vi "Reverse Camera Orientation.vi"(0 "P1X":dbl[](array[numeric]), 1 "P1Y":dbl[](array[numeric]), 2 "P2X":dbl[](array[numeric]), 3 "P2Y":dbl[](array[numeric]), 4 "P3X":dbl[](array[numeric]), 5 "P3Y":dbl[](array[numeric]), 6 "Apply Transform?":bool, 7 "Calibration Data":T1 {"y" format="%.2f"; "z" format="%.2f"; "theta" format="%.2f"; "phi" format="%.2f"; "d" format="%.2f"}, 8 "Stored Camera Orientation":enum16{"Horizontal", "Vertical"}(ring), 10 "Eye":enum16{"Right", "Left"}(ring)=enum."Left") -> (13 "Calibration Data out":T1 {"y" format="%.2f"; "z" format="%.2f"; "theta" format="%.2f"; "phi" format="%.2f"; "d" format="%.2f"}, 14 "P1X out":dbl[](array[numeric]), 15 "P1Y out":dbl[](array[numeric]), 16 "P2X out":dbl[](array[numeric]), 17 "P2Y out":dbl[](array[numeric]), 18 "P3X out":dbl[](array[numeric]), 19 "P3Y out":dbl[](array[numeric]))   [LabVIEW 2016]
doc: "Author: William Figtree\nDate: 7/02/2016\nDescription:\nVI reverse the camera orientation selected during aquisition by transforming the X and Y pixel coordinates.s"
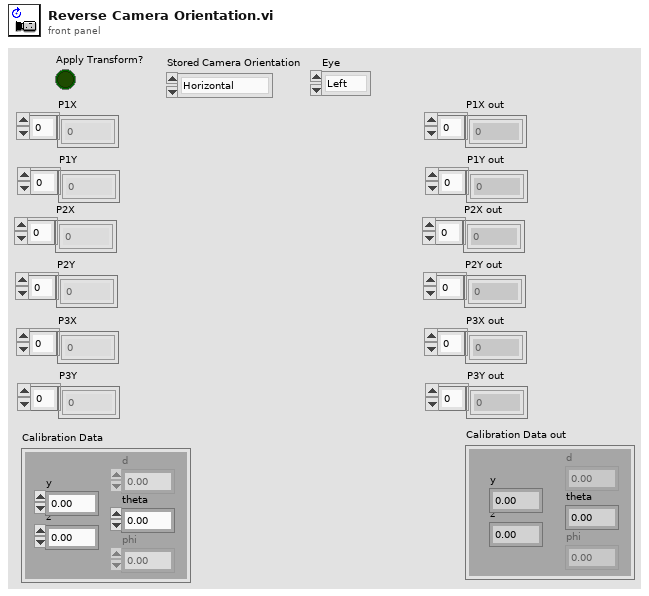
[diagram p1: front panel]
types:
  T1 = cluster{"d":dbl, "phi":dbl, "theta":dbl, "z":dbl, "y":dbl}
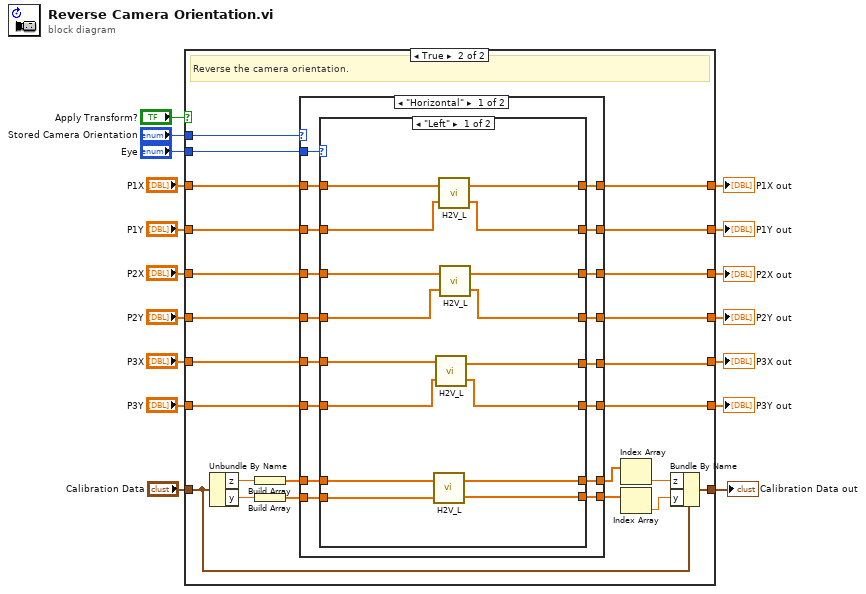
[diagram p0: block diagram]
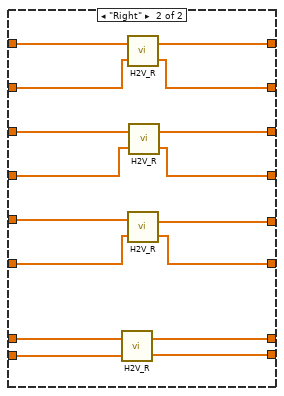
[diagram p3: hidden frame]
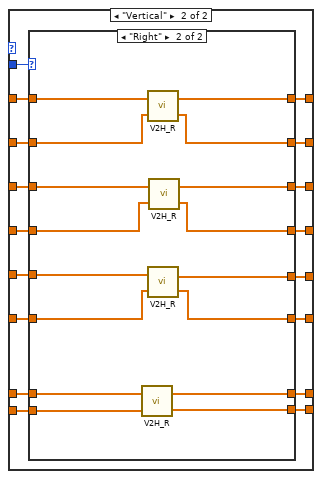
[diagram p4: hidden frame]
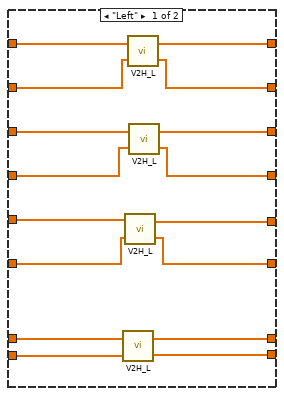
[diagram p5: hidden frame]
diagram:
  n1 = case shown="True" "Apply Transform?" {
    tunnel: "Calibration Data" -> [w18 w48]
    tunnel: [w18 w47] -> w16
    tunnel: "Stored Camera Orientation" -> [_ w46]
    tunnel: "Eye" -> [_ w45]
    tunnel: "P1X" -> [w24 w44]
    tunnel: "P1Y" -> [w23 w43]
    tunnel: "P2X" -> [w22 w42]
    tunnel: "P2Y" -> [w21 w41]
    tunnel: "P3X" -> [w20 w40]
    tunnel: "P3Y" -> [w19 w39]
    tunnel: [w24 w38] -> w6
    tunnel: [w23 w37] -> w5
    tunnel: [w22 w36] -> w4
    tunnel: [w21 w35] -> w3
    tunnel: [w20 w34] -> w2
    tunnel: [w19 w33] -> w1
    frame False {
      # "Do nothing."
    }
    frame True {
      # "Reverse the camera orientation."
      n2 = Unbundle By Name(w48) -> ("z"=w32:dbl, "y"=w31:dbl)
      n3 = Build Array(w32) -> (w30:dbl[])
      n4 = Build Array(w31) -> (w29:dbl[])
      n5 = case shown="\"Horizontal\"" w46 {
        tunnel: w45 -> [w65 w114]
        tunnel: w44 -> [w64 w113]
        tunnel: w43 -> [w63 w112]
        tunnel: w42 -> [w62 w111]
        tunnel: w41 -> [w61 w110]
        tunnel: w40 -> [w60 w109]
        tunnel: w39 -> [w59 w108]
        tunnel: w30 -> [w58 w107]
        tunnel: w29 -> [w57 w106]
        tunnel: [w56 w105] -> w38
        tunnel: [w55 w104] -> w37
        tunnel: [w54 w103] -> w36
        tunnel: [w53 w102] -> w35
        tunnel: [w52 w101] -> w34
        tunnel: [w51 w100] -> w33
        tunnel: [w50 w99] -> w28
        tunnel: [w49 w98] -> w27
        frame "Horizontal" {
          n6 = case shown="\"Left\"" w65 {
            tunnel: w64 -> [w81 w97]
            tunnel: w63 -> [w80 w96]
            tunnel: w62 -> [w77 w93]
            tunnel: w61 -> [w76 w92]
            tunnel: w60 -> [w73 w89]
            tunnel: w59 -> [w72 w88]
            tunnel: w58 -> [w69 w85]
            tunnel: w57 -> [w68 w84]
            tunnel: [w79 w94] -> w56
            tunnel: [w78 w95] -> w55
            tunnel: [w75 w90] -> w54
            tunnel: [w74 w91] -> w53
            tunnel: [w71 w86] -> w52
            tunnel: [w70 w87] -> w51
            tunnel: [w67 w82] -> w50
            tunnel: [w66 w83] -> w49
            frame "Left" {
              n7 = call "H2V_L.vi"("YL in"=w68, "XL in"=w69) -> ("YL out"=w66:dbl[], "XL out"=w67:dbl[])
              n8 = call "H2V_L.vi"("YL in"=w72, "XL in"=w73) -> ("YL out"=w70:dbl[], "XL out"=w71:dbl[])
              n9 = call "H2V_L.vi"("YL in"=w80, "XL in"=w81) -> ("YL out"=w78:dbl[], "XL out"=w79:dbl[])
              n10 = call "H2V_L.vi"("YL in"=w76, "XL in"=w77) -> ("YL out"=w74:dbl[], "XL out"=w75:dbl[])
            }
            frame "Right" {
              n11 = call "H2V_R.vi"("YL in"=w84, "XL in"=w85) -> ("YL out"=w83:dbl[], "XL out"=w82:dbl[])
              n12 = call "H2V_R.vi"("YL in"=w96, "XL in"=w97) -> ("YL out"=w95:dbl[], "XL out"=w94:dbl[])
              n13 = call "H2V_R.vi"("YL in"=w88, "XL in"=w89) -> ("YL out"=w87:dbl[], "XL out"=w86:dbl[])
              n14 = call "H2V_R.vi"("YL in"=w92, "XL in"=w93) -> ("YL out"=w91:dbl[], "XL out"=w90:dbl[])
            }
          }
        }
        frame "Vertical" {
          n15 = case shown="\"Right\"" w114 {
            tunnel: w113 -> [w130 w146]
            tunnel: w112 -> [w129 w145]
            tunnel: w111 -> [w126 w142]
            tunnel: w110 -> [w125 w141]
            tunnel: w109 -> [w122 w138]
            tunnel: w108 -> [w121 w137]
            tunnel: w107 -> [w118 w134]
            tunnel: w106 -> [w117 w133]
            tunnel: [w128 w143] -> w105
            tunnel: [w127 w144] -> w104
            tunnel: [w124 w139] -> w103
            tunnel: [w123 w140] -> w102
            tunnel: [w120 w135] -> w101
            tunnel: [w119 w136] -> w100
            tunnel: [w116 w131] -> w99
            tunnel: [w115 w132] -> w98
            frame "Left" {
              n16 = call "V2H_L.vi"("YL in"=w117, "XL in"=w118) -> ("YL out"=w115:dbl[], "XL out"=w116:dbl[])
              n17 = call "V2H_L.vi"("YL in"=w121, "XL in"=w122) -> ("YL out"=w119:dbl[], "XL out"=w120:dbl[])
              n18 = call "V2H_L.vi"("YL in"=w129, "XL in"=w130) -> ("YL out"=w127:dbl[], "XL out"=w128:dbl[])
              n19 = call "V2H_L.vi"("YL in"=w125, "XL in"=w126) -> ("YL out"=w123:dbl[], "XL out"=w124:dbl[])
            }
            frame "Right" {
              n20 = call "V2H_R.vi"("YL in"=w133, "XL in"=w134) -> ("YL out"=w132:dbl[], "XL out"=w131:dbl[])
              n21 = call "V2H_R.vi"("YL in"=w145, "XL in"=w146) -> ("YL out"=w144:dbl[], "XL out"=w143:dbl[])
              n22 = call "V2H_R.vi"("YL in"=w137, "XL in"=w138) -> ("YL out"=w136:dbl[], "XL out"=w135:dbl[])
              n23 = call "V2H_R.vi"("YL in"=w141, "XL in"=w142) -> ("YL out"=w140:dbl[], "XL out"=w139:dbl[])
            }
          }
        }
      }
      n24 = Index Array(array=w28) -> (element=w25:dbl)  [unwired: 1 in]
      n25 = Index Array(array=w27) -> (element=w26:dbl)  [unwired: 1 in]
      n26 = Bundle By Name(cluster=w48, "z"=w25, "y"=w26) -> (w47:T1)
    }
  }
  "P1X out" <- w6
  "P1Y out" <- w5
  "P2X out" <- w4
  "P2Y out" <- w3
  "P3X out" <- w2
  "P3Y out" <- w1
  "Calibration Data out" <- w16
